vi "Read Version Control.vi"(4 "error in (no error)":errorcluster, 6 "Version Control Name (\"Version\")":string="Version", 7 "Path to Version Global (empty)":path) -> (0 "error out":errorcluster, 3 "Version":T1 {"Build Date/Time" format="%<%X\n%x>T"})   [LabVIEW 2011]
uses:
  OGAB Version.ctl
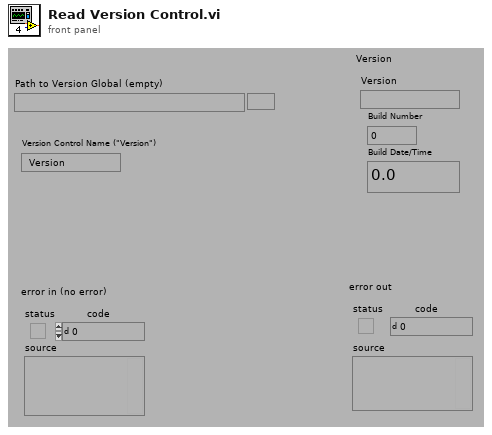
[diagram p1: front panel]
types:
  T1 = typedef "OGAB Version.ctl" = cluster{"Version":string, "Build Number":u32, "Build Date/Time":dbl}
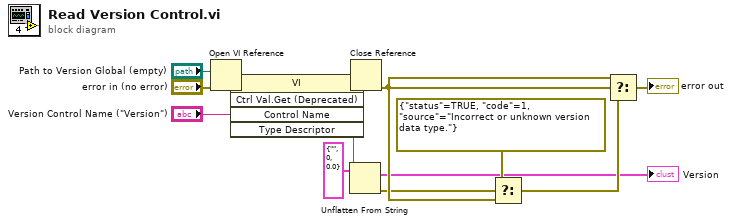
[diagram p0: block diagram]
diagram:
  n1 = Open VI Reference(vi path="Path to Version Global (empty)", error in (no error)="error in (no error)") -> (vi reference=w12:refnum<vi>, error out=w13:errorcluster)  [unwired: 4 out]
  n2 = invoke class="VI" method="Ctrl Val.Get (Deprecated)"(reference=w12, error in=w13, "Control Name"="Version Control Name (\"Version\")") -> (reference out=w8:refnum<vi>, error out=w9:errorcluster, "Get Control Value"=w10:string)  [unwired: 2 in, 2 out]
  n3 = Unflatten From String(type=T1 {"Version"="", "Build Number"=0, "Build Date/Time"=0.0} ("Version"), binary string=w10) -> (value=→"Version":T1, error out=w1:errorcluster)  [unwired: 1 in, 3 out]
  n4 = Close Reference(reference=w8, error in (no error)=w9) -> (error out=w4:errorcluster)
  n5 = Select(t=errorcluster {"status"=TRUE, "code"=1, "source"="Incorrect or unknown version data type."} ("error out"), s=w1, f=w4) -> (s? t:f=w3:errorcluster)
  n6 = Select(t=w4, s=w4, f=w3) -> (s? t:f=→"error out":errorcluster)
